vi "Write PW Limits.vi"(8 "error in (no error)":errorcluster, 9 "low pw (us)":dbl, 10 "high pw (us)":dbl, 11 "Controller in":refnum<class "Controller.lvclass">) -> (0 "error out":errorcluster, 3 "Controller out":refnum<class "Controller.lvclass">)   [LabVIEW 2020, in "Controller.lvclass"]
uses:
  Controller.lvclass
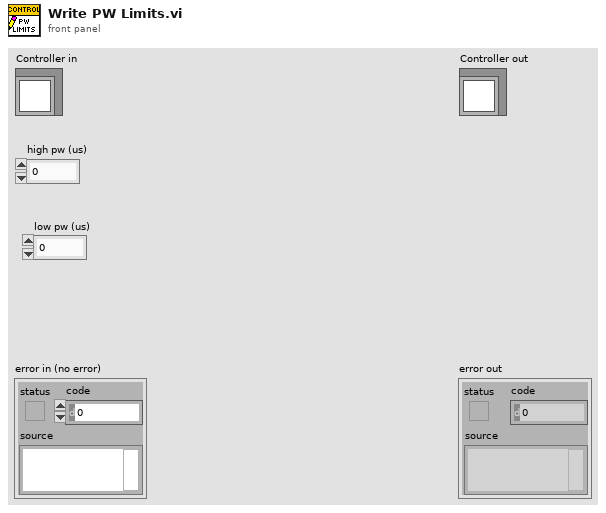
[diagram p1: front panel]
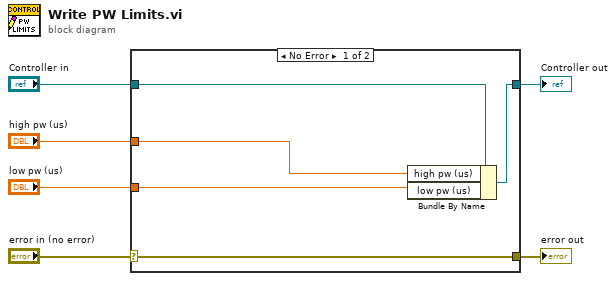
[diagram p0: block diagram]
diagram:
  n1 = case shown="No Error" "error in (no error)" {
    selector: "error in (no error)" -> [w11 w12]
    tunnel: [w11 w12] -> w5
    tunnel: [w9 w13] -> w3
    tunnel: "Controller in" -> [w10 w13]
    tunnel: "high pw (us)" -> [w8 _]
    tunnel: "low pw (us)" -> [w7 _]
    frame No Error {
      n2 = Bundle By Name(cluster=w10, "high pw (us)"=w8, "low pw (us)"=w7) -> (w9:refnum<class "Controller.lvclass">)
    }
    frame Error {
    }
  }
  "error out" <- w5
  "Controller out" <- w3
